vi "Convert 2D to 1D.vi"   [LabVIEW 2014]
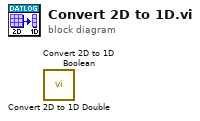
[diagram p0: block diagram]
diagram:
  n1 = call "Convert 2D to 1D Double.vi"() -> ()  [unwired: 10 in, 2 out]
  n2 = call "Convert 2D to 1D Boolean.vi"() -> ()  [unwired: 10 in, 2 out]
